vi "ABB convert dropdown.vi"(7 "Mode":enum16{"# 2 string", "string 2 #"}(ring), 9 "String in":string, 10 "# in":i32, 11 "Strings":string[](array[string])) -> (1 "String out":string, 2 "#out":i32)   [LabVIEW 2017]
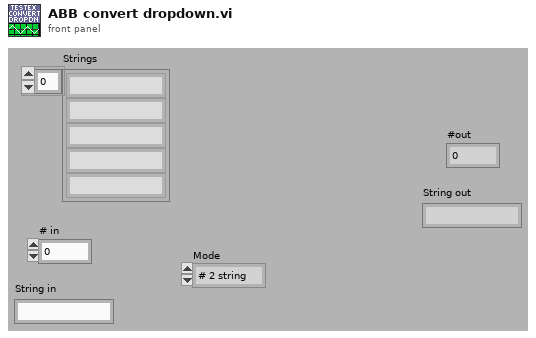
[diagram p1: front panel]
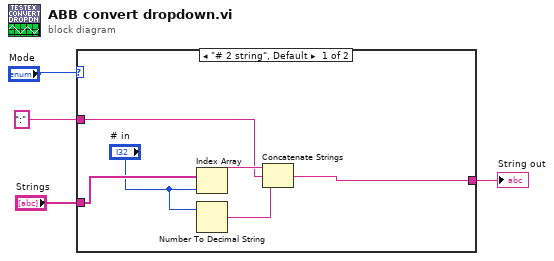
[diagram p0: block diagram]
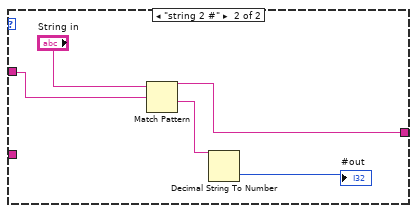
[diagram p2: hidden frame]
diagram:
  n1 = case shown="\"# 2 string\", Default" "Mode" {
    tunnel: "Strings" -> [w10 _]
    tunnel: ":" ("string") -> [w6 w14]
    tunnel: [w5 w13] -> w1
    frame "# 2 string", Default {
      n2 = Index Array(array=w10, index="# in") -> (element=w9:string)
      n3 = Number To Decimal String(number="# in") -> (decimal integer string=w7:string)  [unwired: 1 in]
      n4 = Concatenate Strings(w9, w6, w7) -> (w5:string)
    }
    frame "string 2 #" {
      n5 = Match Pattern(string="String in", regular expression=w14) -> (before substring=w13:string, after substring=w12:string)  [unwired: 1 in, 2 out]
      n6 = Decimal String To Number(string=w12) -> (number=→"#out":i32)  [unwired: 2 in, 1 out]
    }
  }
  "String out" <- w1
